vi "Vehicle out of Position Update.vi"(8 "error in (no error)":errorcluster, 10 "Vehicle ouf ot Position":bool, 11 "Car Position Simulation View Definition in":refnum<class "Car Position Simulation View Definition.lvclass">) -> (0 "error out":errorcluster, 3 "Car Position Simulation View Definition out":refnum<class "Car Position Simulation View Definition.lvclass">)   [LabVIEW 2019, in "Car Position Simulation View Definition.lvclass"]
uses:
  <vilib>/gpm_packages/@cs/Car-wash/Source/Car Position Simulation View Definition/Car Position Simulation View Definition/Car Position Simulation View Definition.lvclass
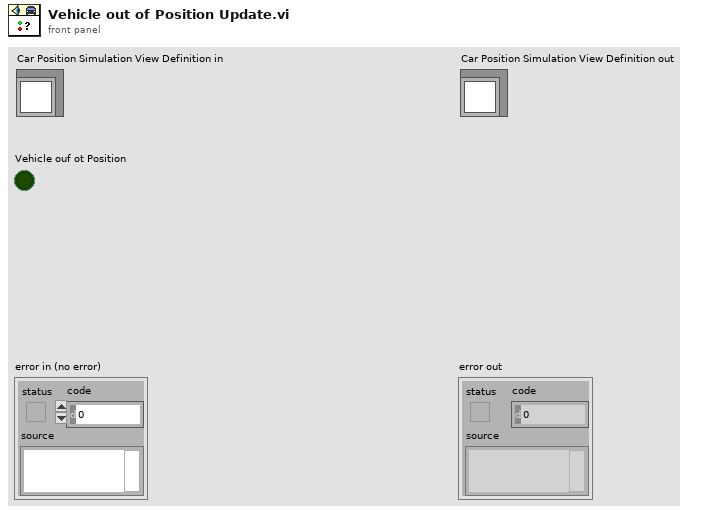
[diagram p1: front panel]
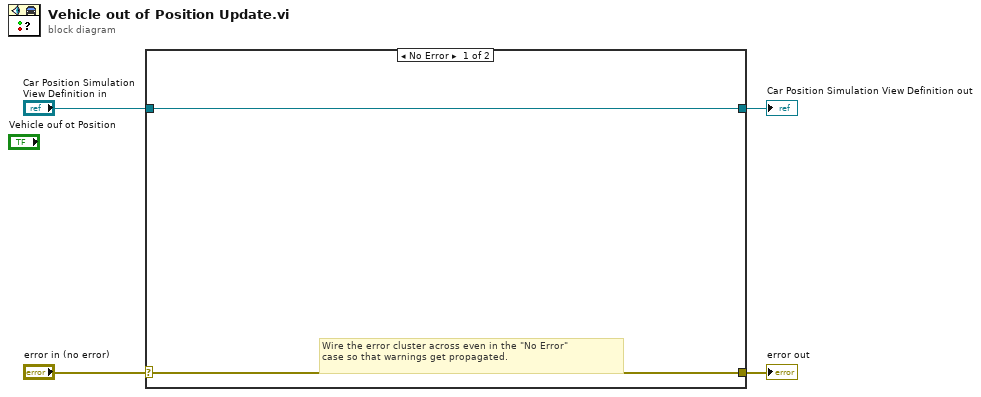
[diagram p0: block diagram]
diagram:
  n1 = case shown="No Error" "error in (no error)" {
    selector: "error in (no error)" -> [w5 w8]
    tunnel: [w5 w8] -> w3
    tunnel: [w6 w7] -> w1
    tunnel: "Car Position Simulation View Definition in" -> [w6 w7]
    frame No Error {
      # "Wire the error cluster across even in the \"No Error\"\ncase so that warnings get propagated."
    }
    frame Error {
    }
  }
  "error out" <- w3
  "Car Position Simulation View Definition out" <- w1
